vi "Destroy.vi"(8 "error in (no error)":errorcluster, 11 "I2C Bus in":refnum<class "Mock I2C Bus.lvclass">) -> (0 "error out":errorcluster)   [LabVIEW 2020, in "Mock I2C Bus.lvclass"]
uses:
  Mock I2C Bus.lvclass
  C:/Program Files (x86)/National Instruments/LabVIEW 2020/vi.lib/Astemes/LMock/Mock.lvclass
  <vilib>/Astemes/LMock/Mock.lvclass
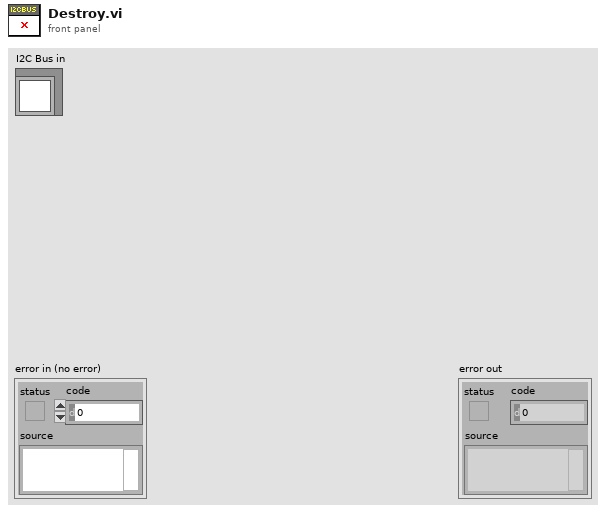
[diagram p1: front panel]
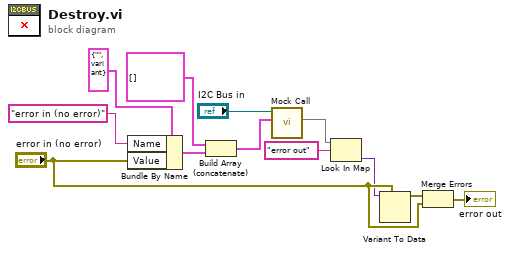
[diagram p0: block diagram]
diagram:
  n1 = Bundle By Name(cluster=cluster{"Name":string, "Value":variant} {"Name"="", "Value"=variant} ("element"), "Name"="error in (no error)", "Value"="error in (no error)") -> (w1:cluster{"Name":string, "Value":variant})
  n2 = Build Array (concatenate)(cluster{"Name":string, "Value":variant}[] [] ("Control Values"), w1) -> (w10:cluster{"Name":string, "Value":variant}[])
  n3 = call <vilib>:"Mock Call.vi"("Control Values"=w10, "Mock In"="I2C Bus in") -> ("Return Values"=w8:map{string, variant})  [unwired: 8 in, 1 out]
  n4 = Look In Map(map=w8, key="error out") -> (value=w6:variant)  [unwired: 1 in, 1 out]
  n5 = Variant To Data(type="error in (no error)", Variant=w6) -> (data=w5:errorcluster)  [unwired: 1 in, 1 out]
  n6 = Merge Errors(w5, "error in (no error)") -> (→"error out":errorcluster)
